vi "Memory.Pointer.Move Block.Safe.vi"(0 "src Pointer in":refnum<class "Memory.Pointer.Void.lvclass">, 1 "length":u64 format="%d bytes", 5 "dst Pointer in":refnum<class "Memory.Pointer.Void.lvclass">, 7 "src offset (0)":u64 format="%d bytes", 9 "dst offset (0)":u64 format="%d bytes", 11 "error in (no error)":errorcluster) -> (4 "src Pointer out":refnum<class "Memory.Pointer.Void.lvclass">, 6 "dst Pointer out":refnum<class "Memory.Pointer.Void.lvclass">, 15 "error out":errorcluster)   [LabVIEW 2016, in "Memory.Pointer.Void.lvclass"]
uses:
  Memory.Pointer.Void.lvclass
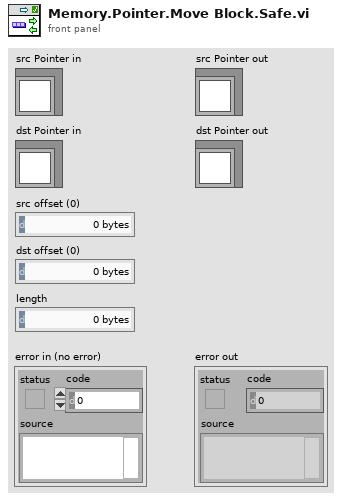
[diagram p1: front panel]
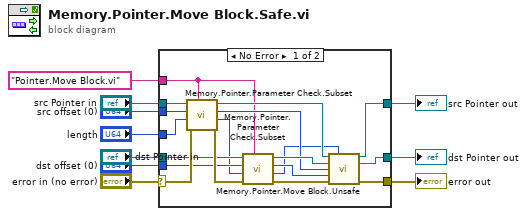
[diagram p0: block diagram]
diagram:
  n1 = case shown="No Error" "error in (no error)" {
    selector: "error in (no error)" -> [w28 w31]
    tunnel: "src Pointer in" -> [w26 w29]
    tunnel: "dst Pointer in" -> [w25 w30]
    tunnel: [w22 w29] -> w8
    tunnel: [w21 w30] -> w7
    tunnel: "length" -> [w20 _]
    tunnel: "src offset (0)" -> [w19 _]
    tunnel: "dst offset (0)" -> [w18 _]
    tunnel: [w13 w31] -> w3
    tunnel: "Pointer.Move Block.vi" ("calling vi name") -> [w12 _]
    frame No Error {
      n2 = call "Memory.Pointer.Parameter Check.Subset.vi"("calling vi name"=w12, "error in (no error)"=w28, "length"=w20, "offset"=w19, "Pointer in"=w26) -> ("error out"=w27:errorcluster, "length out"=w15:u64, "offset out"=w16:u64, "Pointer out"=w23:refnum<class "Memory.Pointer.Void.lvclass">)  [unwired: 3 in]
      n3 = call "Memory.Pointer.Parameter Check.Subset.vi"("calling vi name"=w12, "error in (no error)"=w27, "length"=w15, "offset"=w18, "Pointer in"=w25) -> ("error out"=w11:errorcluster, "length out"=w14:u64, "offset out"=w17:u64, "Pointer out"=w24:refnum<class "Memory.Pointer.Void.lvclass">)  [unwired: 3 in]
      n4 = call "Memory.Pointer.Move Block.Unsafe.vi"("src Pointer in"=w23, "length"=w14, "dst Pointer in"=w24, "src offset (0)"=w16, "dst offset (0)"=w17, "error in (no error)"=w11) -> ("src Pointer out"=w22:refnum<class "Memory.Pointer.Void.lvclass">, "dst Pointer out"=w21:refnum<class "Memory.Pointer.Void.lvclass">, "error out"=w13:errorcluster)  [unwired: 7 in]
    }
    frame Error {
    }
  }
  "error out" <- w3
  "src Pointer out" <- w8
  "dst Pointer out" <- w7
